vi "Mp285Control2.vi"() -> ()   [LabVIEW 2011]
uses:
  SerialController/Serial Controller.lvclass
panel:
  in  "Read Pos":bool
  out "Moving":bool
  out "Move":bool
  out "Relative movement":dbl[](array[numeric])
  out "X-Y":picture
  out "Z":picture
  out "T button?":bool
  in  "Max Step":dbl
  in  "Set Relative":bool
  in  "Absolute":bool caption="Relative"
  in  "Run":bool
  out "X                  Y                 Z":dbl[](array[numeric])=[0.0, 0.0, 5.0] caption="Absolute Position"
  # "Position"
  # "Motor Control"
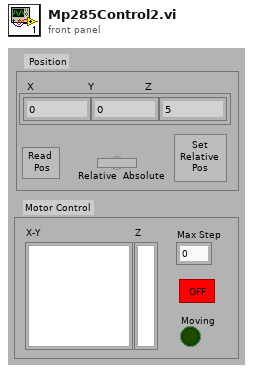
[diagram p1: front panel]
types:
  T1 = cluster{"left":i16, "top":i16, "right":i16, "bottom":i16}
  T2 = cluster{"Width":u16, "Style":enum32{"Solid", "Dash", "Dot", "DashDot", "DashDotDot"}}
  T3 = typedef "LVMouseTypeDef.ctl" = cluster{"Mouse Position":cluster{"X":i32, "Y":i32}, "Mouse Modifiers":cluster{"Button Down":bool, "Shift Mod":bool, "Menu Mod":bool, "Option Mod":bool}}
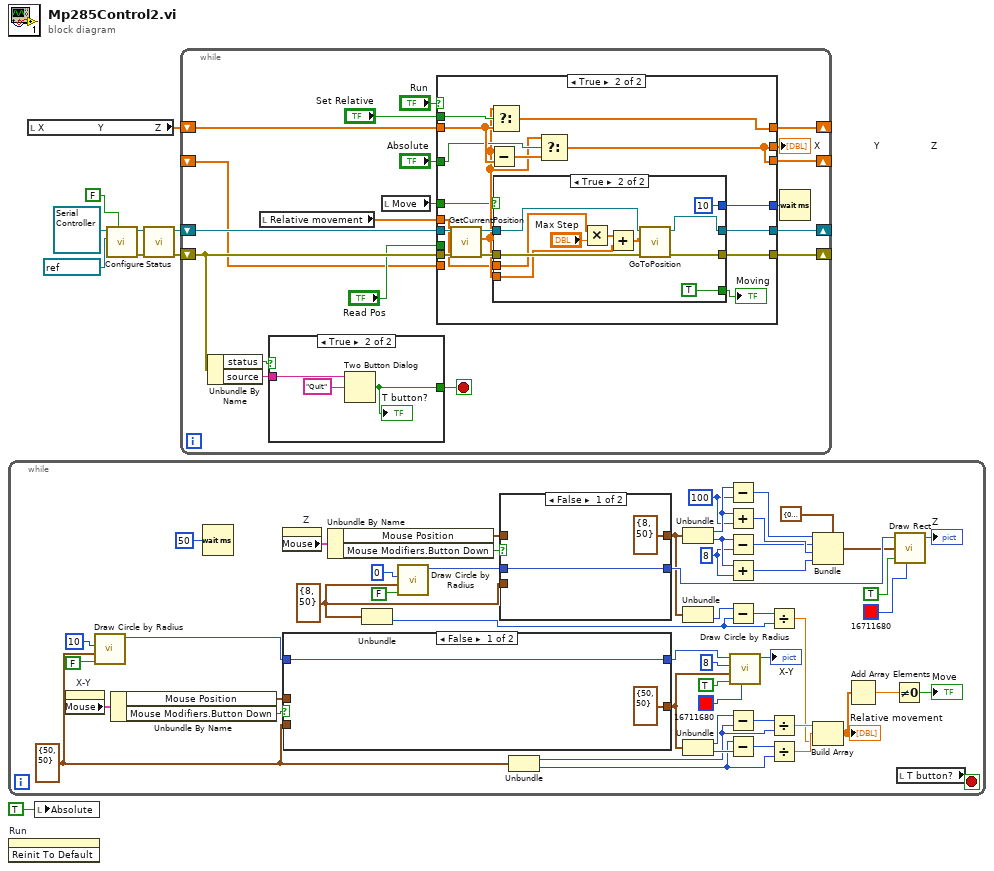
[diagram p0: block diagram]
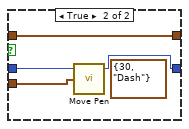
[diagram p2: hidden frame]
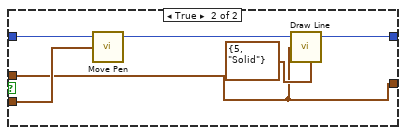
[diagram p3: hidden frame]
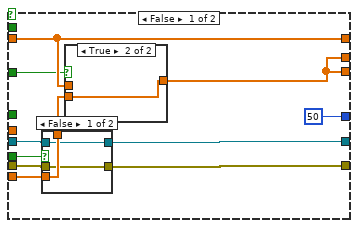
[diagram p5: hidden frame]
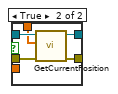
[diagram p6: hidden frame]
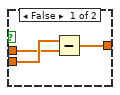
[diagram p7: hidden frame]
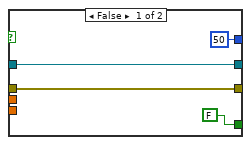
[diagram p8: hidden frame]
diagram:
  n1 = while {
    stop <- w61 stop-if-true
    w20 = 100
    w25 = i16 8 ("radius")
    w32 = cluster{"horizontal":i16, "vertical":i16} {"horizontal"=8, "vertical"=50} ("pixel center")
    w49 = cluster{"horizontal":i16, "vertical":i16} {"horizontal"=50, "vertical"=50} ("pixel center")
    n2 = property on="X-Y" class="Pict"() -> ("Mouse"=w57:T3)  [unwired: 2 in, 2 out]
    n3 = call <vilib>:"Draw Circle by Radius.vi"("fill?(F)"=FALSE, "pixel center"=w49, "radius"=i16 10) -> ("new picture"=w58:picture)  [unwired: 8 in]
    n4 = Unbundle By Name(w57) -> ("Mouse Position"=w50:cluster{"X":i32, "Y":i32}, "Mouse Modifiers.Button Down"=w56:bool)
    n5 = Wait (ms)(milliseconds to wait=u32 50) -> ()  [unwired: 1 out]
    n6 = property on="Z" class="Pict"() -> ("Mouse"=w39:T3)  [unwired: 2 in, 2 out]
    n7 = case shown="False" w56 {
      tunnel: w58 -> [w69 w72]
      tunnel: w50 -> [_ w71]
      tunnel: [w69 w70] -> w51
      tunnel: w49 -> [_ w74]
      tunnel: [cluster{"X":i32, "Y":i32} {"X"=50, "Y"=50} ("Mouse Pos") w71] -> w47
      frame False {
      }
      frame True {
        n8 = call <vilib>:"Move Pen.vi"("new position"=w74, "picture"=w72) -> ("new picture"=w75:picture)  [unwired: 3 in]
        n9 = call <vilib>:"Draw Line.vi"("picture"=w75, "end point"=w71, "pen"=T2 {"Width"=5, "Style"=enum."Solid"}) -> ("new picture"=w70:picture)  [unwired: 6 in]
      }
    }
    n10 = Unbundle By Name(w39) -> ("Mouse Position"=w33:cluster{"X":i32, "Y":i32}, "Mouse Modifiers.Button Down"=w38:bool)
    n11 = Unbundle(w32) -> ("vertical"=w11:i16)  [unwired: 1 out]
    n12 = call <vilib>:"Draw Circle by Radius.vi"("fill?(F)"=FALSE, "pixel center"=w32, "radius"=i16 0) -> ("new picture"=w19:picture)  [unwired: 8 in]
    n13 = case shown="False" w38 {
      tunnel: w33 -> [_ w66]
      tunnel: [w62 w65] -> w34
      tunnel: w32 -> [_ w67]
      tunnel: [cluster{"X":i32, "Y":i32} {"X"=8, "Y"=50} ("Mouse Pos") w66] -> w29
      tunnel: w19 -> [w62 w64]
      frame False {
      }
      frame True {
        (unwired) T2 {"Width"=30, "Style"=enum."Dash"} ("pen")
        n14 = call <vilib>:"Move Pen.vi"("new position"=w67, "picture"=w64) -> ("new picture"=w65:picture)  [unwired: 3 in]
      }
    }
    n15 = Unbundle(w49) -> ("horizontal"=w44:i16, "vertical"=w42:i16)
    n16 = Unbundle(w29) -> ("X"=w27:i32, "Y"=w26:i32)
    n17 = Unbundle(w29) -> ("Y"=w10:i32)  [unwired: 1 out]
    n18 = Unbundle(w47) -> ("X"=w48:i32, "Y"=w46:i32)
    n19 = Subtract(x=w27, y=w20) -> (x-y=w23:i32)
    n20 = Add(x=w27, y=w20) -> (x+y=w24:i32)
    n21 = Subtract(x=w26, y=w25) -> (x-y=w22:i32)
    n22 = Add(x=w26, y=w25) -> (x+y=w21:i32)
    n23 = Subtract(x=w10, y=w11) -> (x-y=w31:i32)
    n24 = Subtract(x=w48, y=w44) -> (x-y=w45:i32)
    n25 = Subtract(x=w42, y=w46) -> (x-y=w43:i32)
    n26 = call <vilib>:"Draw Circle by Radius.vi"("color(black)"=u32 16711680, "fill?(F)"=TRUE, "pixel center"=w47, "radius"=i16 8, "picture"=w51) -> ("new picture"=→"X-Y":picture)  [unwired: 6 in]
    n27 = Divide(x=w31, y=w11) -> (x/y=w16:dbl)
    n28 = Divide(x=w45, y=w44) -> (x/y=w18:dbl)
    n29 = Divide(x=w43, y=w42) -> (x/y=w17:dbl)
    n30 = Bundle(cluster=T1 {"left"=0, "top"=0, "right"=10, "bottom"=10} ("rect"), "left"=w23, "top"=w22, "right"=w24, "bottom"=w21) -> (w28:T1)
    n31 = Build Array(w18, w17, w16) -> (w15:dbl[])
    "Relative movement" <- w15
    n32 = Add Array Elements(numeric array=w15) -> (sum=w14:dbl)
    n33 = Not Equal To 0?(x=w14) -> (x != 0?=→"Move":bool)
    n34 = call <vilib>:"Draw Rect.vi"("picture"=w34, "rect"=w28, "fill?(F)"=TRUE, "color(black)"=u32 16711680) -> ("new picture"=→"Z":picture)  [unwired: 5 in]
    n35 = local read "T button?"() -> (w61:bool)
  }
  n36 = invoke on="Run" class="Bool (strict)" method="Reinit To Default"() -> ()  [unwired: 3 in, 3 out]
  n37 = local read "X                  Y                 Z"() -> (w4:dbl[])
  n38 = local write "Absolute"(TRUE) -> ()
  n39 = call-dynamic "Configure.vi"("Reset"=FALSE, "VISA resource name"=refnum<visa-resource-name> "COM6", "Serial Controller in"=refnum<class "Serial Controller.lvclass"> refnum) -> ("error out"=w8:errorcluster, "Serial Controller out"=w9:refnum<class "Serial Controller.lvclass">)  [unwired: 7 in]
  n40 = call-dynamic "Status.vi"("error in (no error)"=w8, "Serial Controller in"=w9) -> ("error out"=w1:errorcluster, "Serial Controller out"=w2:refnum<class "Serial Controller.lvclass">)  [unwired: 7 in, 1 out]
  n41 = while {
    shift-right: [w91] -> _
    shift-left: w4 -> [w92]
    shift-right: [w83] -> _
    shift-left: w2 -> [w82]
    shift-right: [w84] -> _
    shift-left: w1 -> [w81]
    shift-right: [w77] -> _
    shift-left: _ -> [w76]
    stop <- w85 stop-if-true
    n42 = Unbundle By Name(w81) -> ("status"=w86:bool, "source"=w87:string)
    n43 = local read "Relative movement"() -> (w80:dbl[])
    n44 = case shown="True" w86 {
      tunnel: w87 -> [_ w97]
      tunnel: [_ w95] -> w85
      frame False {
      }
      frame True {
        n45 = Two Button Dialog(message=w97, 2:"Quit" ("T button name (\"OK\")")) -> (T button?=w95:bool)  [unwired: 1 in]
        "T button?" <- w95
      }
    }
    n46 = local read "Move"() -> (w79:bool)
    n47 = case shown="True" "Run" {
      tunnel: w82 -> [w108 w137]
      tunnel: w81 -> [w107 w136]
      tunnel: "Absolute" -> [w104 w128]
      tunnel: w92 -> [w105 w130]
      tunnel: [w105 w132] -> w91
      tunnel: "Set Relative" -> [_ w131]
      tunnel: [w99 w121] -> w89
      tunnel: [u32 50 ("milliseconds to wait") w133] -> w88
      tunnel: w79 -> [_ w126]
      tunnel: w80 -> [_ w125]
      tunnel: [w102 w123] -> w84
      tunnel: [w101 w124] -> w83
      tunnel: "Read Pos" -> [w100 _]
      tunnel: [w99 w121] -> w77
      tunnel: w76 -> [w98 _]
      frame False {
        n48 = case shown="False" w100 {
          tunnel: w108 -> [w110 w116]
          tunnel: w107 -> [w109 w115]
          tunnel: [w111 w114] -> w106
          tunnel: [w109 w113] -> w102
          tunnel: [w110 w112] -> w101
          tunnel: w98 -> [w111 _]
          frame False {
          }
          frame True {
            n49 = call-dynamic "GetCurrentPosition.vi"("error in (no error)"=w115, "Serial Controller in"=w116) -> ("error out"=w113:errorcluster, "Position"=w114:dbl[], "Serial Controller out"=w112:refnum<class "Serial Controller.lvclass">)  [unwired: 6 in, 1 out]
          }
        }
        n50 = case shown="True" w104 {
          tunnel: w106 -> [w118 w120]
          tunnel: [w119 w120] -> w99
          tunnel: w105 -> [w117 _]
          frame False {
            n51 = Subtract(x=w118, y=w117) -> (x-y=w119:dbl[])
          }
          frame True {
          }
        }
      }
      frame True {
        n52 = call-dynamic "GetCurrentPosition.vi"("error in (no error)"=w136, "Serial Controller in"=w137) -> ("error out"=w135:errorcluster, "Position"=w127:dbl[], "Serial Controller out"=w134:refnum<class "Serial Controller.lvclass">)  [unwired: 6 in, 1 out]
        n53 = Subtract(x=w127, y=w130) -> (x-y=w129:dbl[])
        n54 = Select(t=w127, s=w131, f=w130) -> (s? t:f=w132:dbl[])
        n55 = case shown="True" w126 {
          tunnel: w135 -> [w139 w152]
          tunnel: w134 -> [w140 w151]
          tunnel: [u32 50 ("milliseconds to wait") u32 10 ("milliseconds to wait")] -> w133
          tunnel: w127 -> [_ w149]
          tunnel: w125 -> [_ w145]
          tunnel: [w140 w144] -> w124
          tunnel: [w139 w143] -> w123
          tunnel: [FALSE TRUE ("Moving")] -> w122
          frame False {
          }
          frame True {
            n56 = Multiply(x=w145, y="Max Step") -> (x*y=w147:dbl[])
            n57 = Add(x=w147, y=w149) -> (x+y=w146:dbl[])
            n58 = call-dynamic "GoToPosition.vi"("error in (no error)"=w152, "Position"=w146, "Serial Controller in"=w151) -> ("error out"=w143:errorcluster, "Serial Controller out"=w144:refnum<class "Serial Controller.lvclass">)  [unwired: 7 in]
          }
        }
        "Moving" <- w122
        n59 = Select(t=w127, s=w128, f=w129) -> (s? t:f=w121:dbl[])
      }
    }
    "X                  Y                 Z" <- w89
    n60 = Wait (ms)(milliseconds to wait=w88) -> ()  [unwired: 1 out]
  }
